vi "Get IsAsserted.vi"(11 "Leaf.Assertion":refnum<class "Leaf.Assertion.lvclass">) -> (1 "Skipped":bool, 2 "Asserted":bool, 3 "Leaf.Assertion":refnum<class "Leaf.Assertion.lvclass">)   [LabVIEW 2021, in "Bananas.lvlib" / "Leaf.Assertion.lvclass"]
uses:
  Leaf.Assertion.lvclass
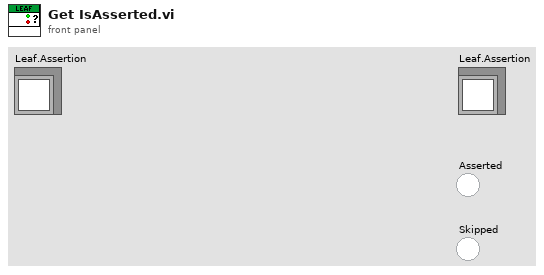
[diagram p1: front panel]
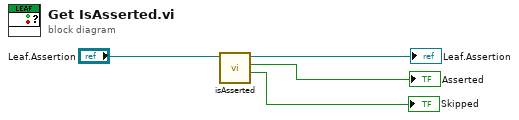
[diagram p0: block diagram]
diagram:
  n1 = call-dynamic "isAsserted.vi"("Leaf.Assertion"="Leaf.Assertion") -> ("Skipped"=→"Skipped":bool, "Asserted"=→"Asserted":bool, "Leaf.Assertion"=→"Leaf.Assertion":refnum<class "Leaf.Assertion.lvclass">)  [unwired: 8 in]
